vi "MGI RWA Delete Section.vi"(8 "Error In":errorcluster, 10 "Section Name":string, 11 "Path":path) -> (0 "Error Out":errorcluster, 2 "Found?":bool)   [LabVIEW 2016]
doc: "Deletes a section in a Read/Write Anything file.\nAuthored by Brandon D. Steele\nsupport@mooregoodideas.com\nwww.mooregoodideas.com\n\nCopyright (c) 2010, Moore Good Ideas, Inc.\n\nAll rights reserved.\n\nRedistribution and use in source and binary forms, with or without modification, are permitted provided that the following conditions are met:\n\n * Redistributions of source code must retain the above copyright notice, this list of conditions and the following disclaimer.\n * Redistributions in binary form must reproduce the above copyright notice, this list of conditions and the following disclaimer in the documentation and/or other materials provided with the distribution.\n * Neither the name of Moore Good Ideas, Inc. nor the names of its contributors may be used to endorse or promote products derived from this software without specific prior written permission.\n\nTHIS SOFTWARE IS PROVIDED BY THE COPYRIGHT HOLDERS AND CONTRIBUTORS \"AS IS\" AND ANY EXPRESS OR IMPLIED WARRANTIES, INCLUDING, BUT NOT LIMITED TO, THE IMPLIED WARRANTIES OF MERCHANTABILITY AND FITNESS FOR A PARTICULAR PURPOSE ARE DISCLAIMED. IN NO EVENT SHALL THE COPYRIGHT OWNER OR CONTRIBUTORS BE LIABLE FOR ANY DIRECT, INDIRECT, INCIDENTAL, SPECIAL, EXEMPLARY, OR CONSEQUENTIAL DAMAGES (INCLUDING, BUT NOT LIMITED TO, PROCUREMENT OF SUBSTITUTE GOODS OR SERVICES; LOSS OF USE, DATA, OR PROFITS; OR BUSINESS INTERRUPTION) HOWEVER CAUSED AND ON ANY THEORY OF LIABILITY, WHETHER IN CONTRACT, STRICT LIABILITY, OR TORT (INCLUDING NEGLIGENCE OR OTHERWISE) ARISING IN ANY WAY OUT OF THE USE OF THIS SOFTWARE, EVEN IF ADVISED OF THE POSSIBILITY OF SUCH DAMAGE."
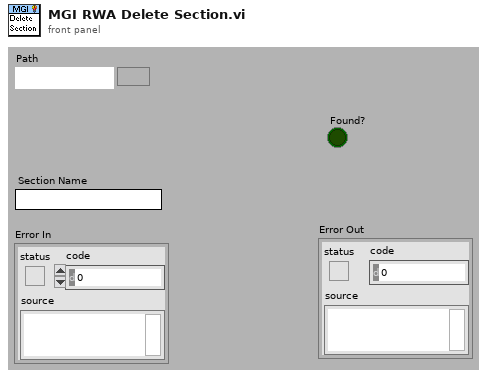
[diagram p1: front panel]
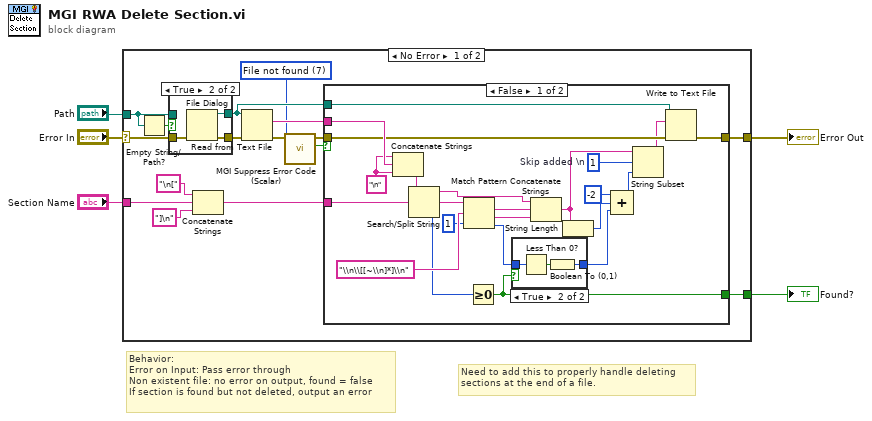
[diagram p0: block diagram]
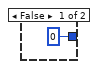
[diagram p2: hidden frame]
diagram:
  # "Need to add this to properly handle deleting\nsections at the end of a file."
  # "Behavior:\nError on Input: Pass error through\nNon existent file: no error on output, found = false\nIf section is found but not deleted, output an error"
  n1 = case shown="No Error" "Error In" {
    selector: "Error In" -> [w7 w55]
    tunnel: "Section Name" -> [w21 _]
    tunnel: [w20 _] -> w4
    tunnel: "Path" -> [w19 _]
    tunnel: [w18 w55] -> w2
    frame No Error {
      w9 = u16 7 items=["No error", "Argument error", "Memory is full", "Out of zone", "End of file", "File already open", "Generic file I/O error", "File not found", "File permission error", "Disk is full", "Duplicate path", "Too many files open", "System feature not enabled", "Resource file not found", "Cannot add resource", "Resource not found", "Image not found", "Image memory error", "Pen does not exist", "Config type invalid", "Config token not found", "Config parse error", "Config memory error", "Bad external code format", "Bad external code offset", "External code not present", "Null window", "Destroy window error", "Null menu", "Print aborted", "Bad print record", "Print driver error", "Windows error during printing", "Memory error during printing", "Print dialog error", "Generic print error", "Invalid device refnum", "Device not found", "Device parameter error", "Device unit error", "Cannot open device", "Device call aborted", "Generic error", "Cancelled by user", "Object ID too low", "Object ID too high", "Object not in heap", "Unknown heap", "Unknown object (invalid DefProc)", "Unknown object (DefProc not in table)", "Message out of range", "Invalid (null) method", "Unknown message", "Manager call not supported", "Bad address", "Network operation in progress", "Network operation timed out", "Connection is busy", "Network attribute not supported", "Network error", "Address in use", "System out of memory", "Connection aborted", "Connection refused", "Not connected", "Already connected", "Connection closed", "Initialization error (interapplication manager)", "Bad occurrence", "Wait on unbound occurrence handler", "Occurrence queue overflow", "Datalog type conflict", "Unused", "Unrecognized type (interapplication manager)", "Memory corrupt", "Failed to make temporary DLL", "Old CIN version", "Drag socket not found", "Failed to load drop-object", "Failed to register OLE object", "Failed to release OLE object", "Format specifier type mismatch", "Unknown format specifier", "Too few format specifiers", "Too many format specifiers", "Scan failed", "Newer CIN version", "OLE Convert", "Runtime menu error", "Password tampered", "Unknown error code"] ("Reserved Error Code (Generic error)")
      n2 = Empty String/Path?(string/path=w19) -> (empty?=w14:bool)
      n3 = case shown="True" w14 {
        tunnel: w7 -> [w50 w54]
        tunnel: [w50 w53] -> w15
        tunnel: [w51 w52] -> w13
        tunnel: w19 -> [w51 _]
        frame False {
        }
        frame True {
          n4 = File Dialog(8:w54) -> (0:w53:errorcluster, 3:w52:path)  [unwired: 8 out]
        }
      }
      n5 = Concatenate Strings("\n[" ("string"), w21, "]\n" ("string")) -> (w12:string)
      n6 = Read from Text File(file (use dialog)=w13, error in=w15) -> (text=w11:string, error out=w10:errorcluster)  [unwired: 4 out]
      n7 = call <userlib>:"MGI Suppress Error Code (Scalar).vi"("Error Code"=w9, "Error In"=w10) -> ("Error Supressed?"=w6:bool, "Error Out"=w8:errorcluster)  [unwired: 4 in]
      n8 = case shown="False" w6 {
        tunnel: [w22 _] -> w20
        tunnel: [w44 w49] -> w18
        tunnel: w13 -> [w43 _]
        tunnel: w12 -> [w42 _]
        tunnel: w11 -> [w41 _]
        tunnel: w8 -> [w37 w49]
        frame False {
          w34 = 1  # Skip added \n
          w32 = "\n" ("string")
          n9 = Concatenate Strings(w32, w41, w32) -> (w36:string)
          n10 = Search/Split String(string=w36, search string/char (-)=w42) -> (substring before match=w39:string, match + rest of string=w38:string, offset of match=w35:i32)  [unwired: 1 in]
          n11 = Match Pattern(string=w38, regular expression="\\n\\[[~\\n]*]\\n", offset (0)=1) -> (match substring=w33:string, after substring=w27:string, offset past match=w24:i32)  [unwired: 1 out]
          n12 = Greater Or Equal To 0?(x=w35) -> (x >= 0?=w22:bool)
          n13 = case shown="True" w22 {
            tunnel: w24 -> [_ w48]
            tunnel: [i16 0 w46] -> w23
            frame False {
            }
            frame True {
              n14 = Less Than 0?(x=w48) -> (x < 0?=w47:bool)
              n15 = Boolean To (0,1)(Boolean=w47) -> (0, 1=w46:i16)
            }
          }
          n16 = Concatenate Strings(w39, w33, w27) -> (w26:string)
          n17 = String Length(string=w26) -> (length=w30:i32)
          n18 = Compound Arithmetic op=ADD(-2 ("value"), w30, w23) -> (w31:i32)
          n19 = String Subset(string=w26, offset (0)=w34, length (rest)=w31) -> (substring=w25:string)
          n20 = Write to Text File(file (use dialog)=w43, text=w25, error in=w37) -> (error out=w44:errorcluster)  [unwired: 3 out]
        }
        frame True {
        }
      }
    }
    frame Error {
    }
  }
  "Error Out" <- w2
  "Found?" <- w4
